vi "TLB Native Dynamic Events ver 0.13 (faulty).vi"() -> ()   [LabVIEW 2018]
uses:
  Labview Training Phase 2/Enum Controls/States for Action Engine.ctl
  TLB Type Definitions/State Type Definitions.ctl
  TLB Type Definitions/Intruction Type Definitions.ctl
  TLB Type Definitions/Encoder cluster.ctl
  TLB Type Definitions/PING CLUSTER.ctl
  <vilib>/Studica/Studica Toolkit/NavX/NavX.lvlib
  <vilib>/Studica/Studica Toolkit/Background/DIO Channel.ctl
  Underlying VI's/NavX VI/navX type def.ctl
  <vilib>/myRIO/Instrument Drivers/Utilities/Utilities.lvlib
  <vilib>/Studica/Studica Toolkit/Background/I2C Channel.ctl
  Underlying VI's/I2C Master VI/I2C MASTER Type Def.ctl
  Experimental VI's/Archived VI's/PID Movement final version Type Def.ctl
  Underlying VI's/I2C Master VI/I2C_MASTER_WRITE_NEW Type Def.ctl
  <vilib>/Studica/Studica Toolkit/NavX/TypeDefs/Flags/Z900_navX_Flags_CalibrationStatusTypeDef.ctl
  <vilib>/Studica/Studica Toolkit/NavX/TypeDefs/Flags/Z900_navX_Flags_OpStatusTypeDef.ctl
panel:
  out "Arduino I2C":errorcluster
  in  "Latch":bool
  in  "y Stepper value":u8
  in  "Arduino mode":T1
  out "Arduino Data":T2
  out "Detect?":bool
  out "Status":T5 {"OP Status" items=["INITIALIZING", "SELFTEST_IN_PROGRESS", "ERROR", "IMU_AUTOCAL_IN_PROGRESS", "NORMAL"]; "Calibration Status" items=["IMU_CAL_STATE_MASK"=3, "IMU_CAL_STATE_INPROGRESS"=0, "IMU_CAL_STATE_ACCUMULATE"=1, "IMU_CAL_STATE_COMPLETE"=2]}
  out "NavX Readings":T6
  out "TASK ENABLE":bool
  out "Rising Edge":bool
  out "Object detected?":bool
  out "navX i2C":errorcluster
  out "Speed & distance":T7
  out "State Logic":T8=enum."Startup"
  out "elements":T9[](array[typedef])
  in  "STOP TASK":bool
  in  "OK Button":bool
  in  "STOP":bool
  out "error out":errorcluster
  out "Action Queue Items":i32
  out "State Logic Queue Items":i32
  out "Action Queues items":string[](array[string])=["Hardware reset", "Software reset", ""]
  out "Action State":string
  # "TLB FRAMEWORK STATUS"
  # "System Health Status Update"
  # "Test Programme written by Calvin Loke    Dated: 28 Aug 2019\nTest Programme revised by Dr Alex See   Dated 30 Aug 2019\n\nProgramme version:   TLB Native Dynamic Events ver 0.04b.vi"
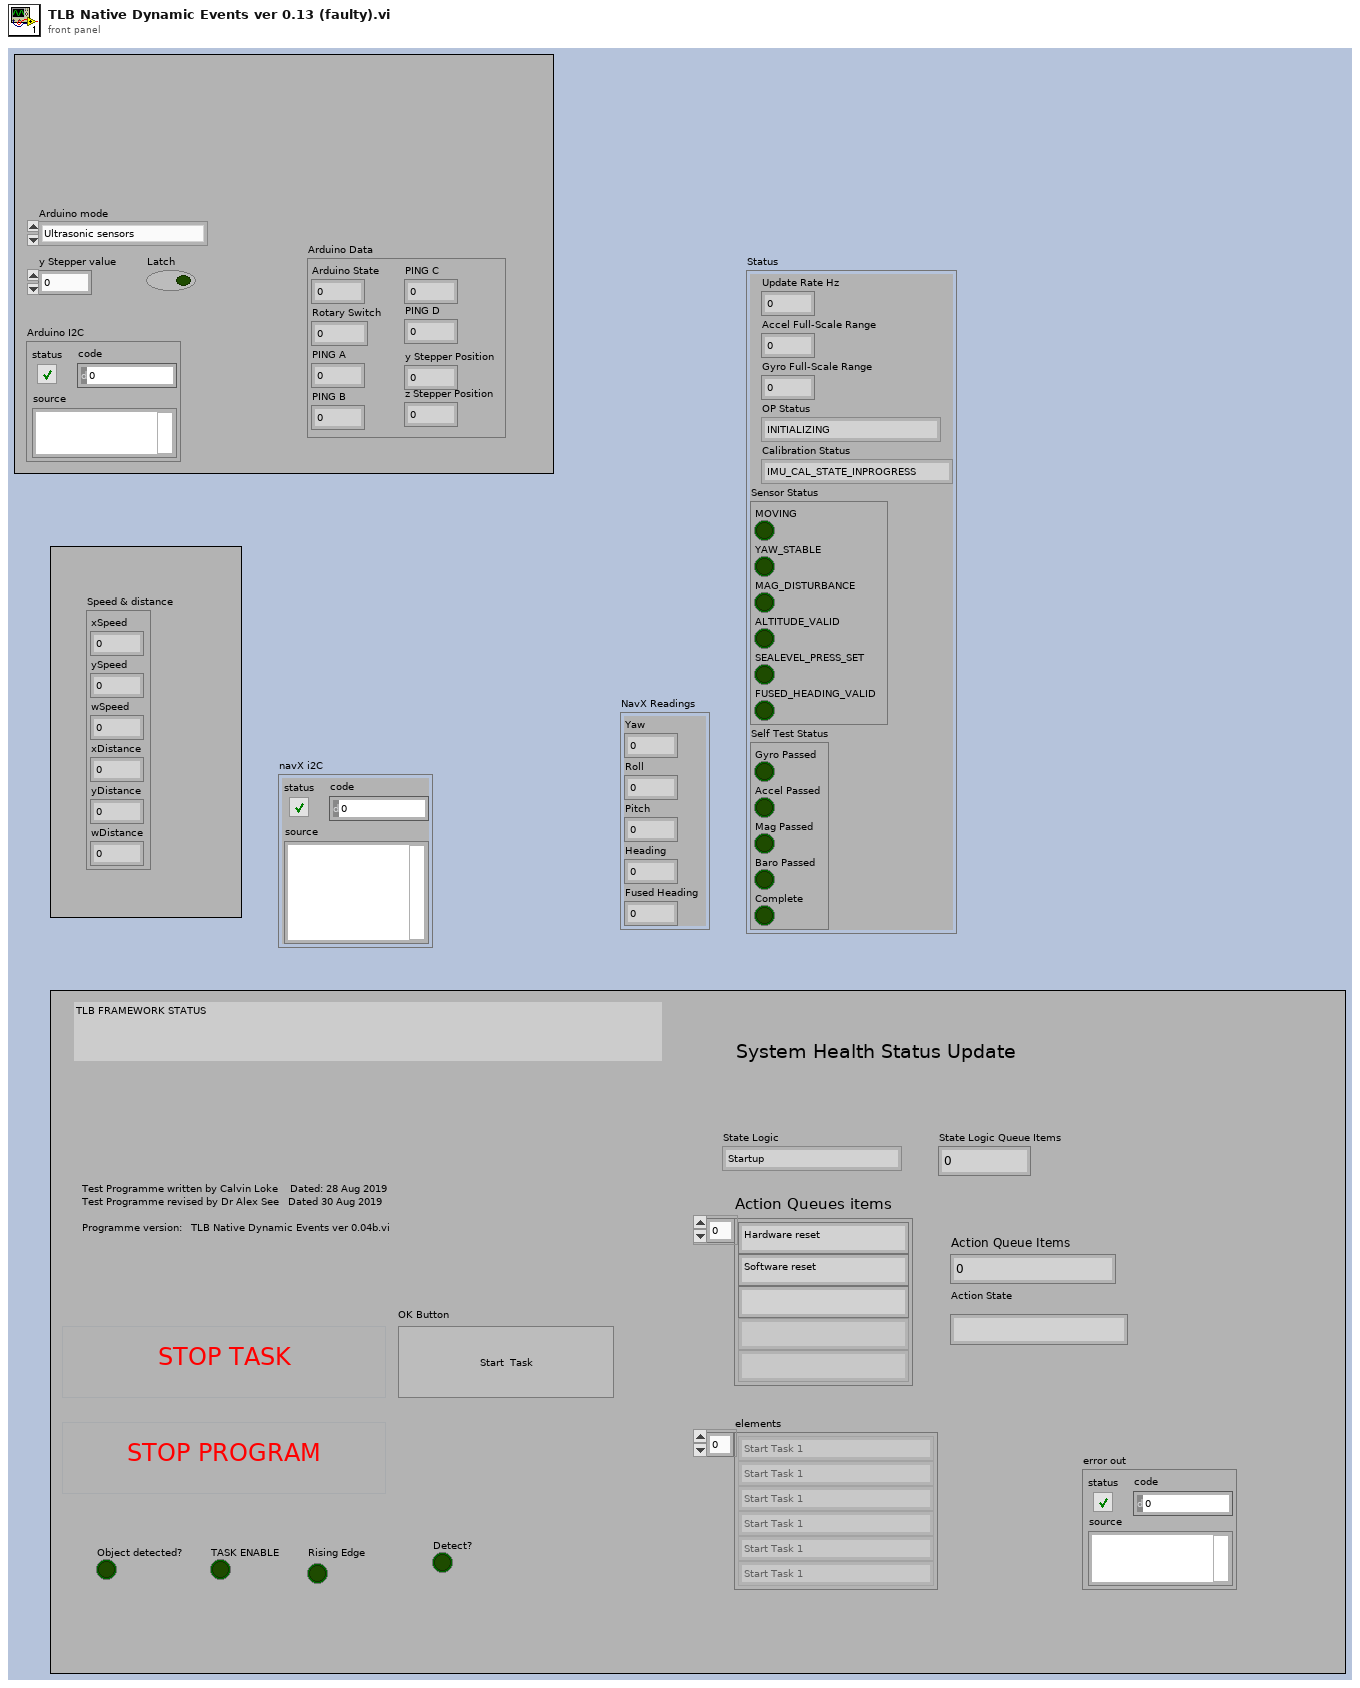
[diagram p1: front panel]
types:
  T1 = typedef "I2C_MASTER_WRITE_NEW Type Def.ctl" = enum16{"Ultrasonic sensors", "Stepper origin", "zStepper 13.3k", "zStepper 13k", "zStepper 12k", "zStepper 11k", "zStepper 10k", "zStepper 9k", "zStepper 8k", "zStepper 7k", "zStepper 6k", "zStepper 5k", "zStepper 4k", "zStepper 3k", "zStepper 2k", "zStepper 1k", "zStepper 900", "zStepper 800", "zStepper 700", "zStepper 600", "zStepper 500", "zStepper 400", "zStepper 300", "zStepper 200", "zStepper 100", "zStepper 0", "yStepper control", "Open Claw", "Close Claw", "Soft Reset"}
  T2 = cluster{"Arduino State":u8, "Rotary Switch":u8, "PING A":u8, "PING B":u8, "PING C":u8, "PING D":u8, "y Stepper Position":u8, "z Stepper Position":u8, "Data Out[8]":u8}
  T3 = typedef "NavX.lvlib/Z900_navX_Flags_OpStatusTypeDef.ctl" = u8
  T4 = typedef "NavX.lvlib/Z900_navX_Flags_CalibrationStatusTypeDef.ctl" = u8
  T5 = cluster{"Update Rate Hz":u8, "Accel Full-Scale Range":u8, "Gyro Full-Scale Range":u16, "OP Status":T3, "Calibration Status":T4, "Sensor Status":cluster{"MOVING":bool, "YAW_STABLE":bool, "MAG_DISTURBANCE":bool, "ALTITUDE_VALID":bool, "SEALEVEL_PRESS_SET":bool, "FUSED_HEADING_VALID":bool}, "Self Test Status":cluster{"Gyro Passed":bool, "Accel Passed":bool, "Mag Passed":bool, "Baro Passed":bool, "Complete":bool}}
  T6 = cluster{"Yaw":dbl, "Roll":dbl, "Pitch":dbl, "Heading":dbl, "Fused Heading":dbl}
  T7 = cluster{"xSpeed":dbl, "ySpeed":dbl, "wSpeed":dbl, "xDistance":dbl, "yDistance":dbl, "wDistance":dbl}
  T8 = typedef "State Type Definitions.ctl" = enum16{"None", "Startup", "Move to Angle", "True Stop", "Idle", "Shutdown", "Task 1A", "Task 1B", "Task 2:Raise Arm", "Task 2:Sensor Mode", "Task 2:Reverse Mode", "Task 3", "Task 4_A", "Task 4_B", "Task 4_C", "Task 4_D", "Task 5A", "Task 5B", "Task 5C", "Task 5D", "Task 5E: POSITION ARM", "Task 5F: ARM GRAB HEIGHT", "Task 5G: CLOSE CLAW", "Task 5H: RAISE ARM", "Task 6_A", "Task 6_B", "Task 7", "Task 8A: RAISE ARM", "Task 8B: MOVE TO BOX", "Task 8C: CAM BURST", "Task 8D: PROCESS IMAGE", "Task 8E: ROBOT ADJUST", "Task 8F: CAM BURST 2", "Task 8G: PROCESS IMAGE 2", "Task 8H: ARM ADJUST", "Task 8I: ARM GRAB HEIGHT", "Task 8J: CLOSE CLAW", "Task 8K: RAISE MY SWORD", "Task 9A: Raise Arm", "Task 9B: Rotate to Angle", "Task 9C: Detect Box", "Task 9D: MOVE FORWARD", "Task 9E: MOVE LEFT", "Task 9F: SCAN IMAGE", "Task 9G: PROCESS COLOUR", "Task 9H: MOVE RIGHT", "Task 9I: SCAN IMAGE", "Task 9J: PROCESS COLOUR", "Task 9K: ROTATE 90 CW", "Task 9L: MOVE FORWARD", "Task 9M: MOVE RIGHT", "Task 9N: SCAN IMAGE", "Task 9O: PROCESS COLOUR", "Task 9P: MOVE RIGHT", "Task 9Q: SCAN IMAGE", "Task 9R: PROCESS COLOUR"}
  T9 = typedef "Intruction Type Definitions.ctl" = enum16{"None", "Start Task 1", "Start Task 2", "Start Task 3", "Start Task 4", "Start Task 5", "Start Task 6", "Start Task 7", "Start Task 8 - BALL", "Start Task 8 - Gel", "Start Task 8 - Pipe", "Start Task 8 - Soap", "Start Task 9", "Start Task A", "Start Task B", "Exit"}
  T10 = typedef "States for Action Engine.ctl" = enum16{"Initialize", "Write", "Read"}
  T11 = typedef "DIO Channel.ctl" = enum16{"Not Connected", "A/DIO1", "A/DIO2", "A/DIO3", "A/DIO4", "A/DIO5", "A/DIO6", "A/DIO7", "A/DIO13", "B/DIO1", "B/DIO2", "B/DIO3", "B/DIO4", "B/DIO5", "B/DIO6", "B/DIO7", "B/DIO13", "C/DIO0", "C/DIO1", "C/DIO2", "C/DIO3", "C/DIO4", "C/DIO5", "C/DIO6", "C/DIO7"}
  T12 = typedef "PING CLUSTER.ctl" = cluster{"PING_A":u8, "PING_B":u8, "PING_C":u8, "PING_D":u8}
  T13 = typedef "Encoder cluster.ctl" = cluster{"xDistance":dbl, "yDistance":dbl, "wDistance":dbl}
  T14 = typedef "I2C Channel.ctl" = enum16{"Not Connected", "A", "B"}
  T15 = typedef "navX type def.ctl" = enum16{"Get i2C reference", "Read Values", "Zero Yaw"}
  T16 = typedef "State Type Definitions.ctl" = enum16{"None", "Startup", "Move to Angle", "True Stop", "Idle", "Shutdown", "Task 1", "Task 2:Raise Arm", "Task 2:Sensor Mode", "Task 2:Reverse Mode", "Task 3", "Task 4_A", "Task 4_B", "Task 4_C", "Task 4_D", "Task 5A: ARM CAM HEIGHT", "Task 5B: MOVE TO BOX", "Task 5C: CAM BURST", "Task 5D: PROCESS IMAGE", "Task 5E: POSITION ARM", "Task 5F: ARM GRAB HEIGHT", "Task 5G: CLOSE CLAW", "Task 5H: RAISE ARM", "Task 6_A", "Task 6_B", "Task 7", "Task 8A: RAISE ARM", "Task 8B: MOVE TO BOX", "Task 8C: CAM BURST", "Task 8D: PROCESS IMAGE", "Task 8E: ROBOT ADJUST", "Task 8F: CAM BURST 2", "Task 8G: PROCESS IMAGE 2", "Task 8H: ARM ADJUST", "Task 8I: ARM GRAB HEIGHT", "Task 8J: CLOSE CLAW", "Task 8K: RAISE MY SWORD", "Task 9A: Raise Arm", "Task 9B: Rotate to Angle", "Task 9C: Detect Box", "Task 9D: MOVE FORWARD", "Task 9E: MOVE LEFT", "Task 9F: SCAN IMAGE", "Task 9G: PROCESS COLOUR", "Task 9H: MOVE RIGHT", "Task 9I: SCAN IMAGE", "Task 9J: PROCESS COLOUR", "Task 9K: ROTATE 90 CW", "Task 9L: MOVE FORWARD", "Task 9M: MOVE RIGHT", "Task 9N: SCAN IMAGE", "Task 9O: PROCESS COLOUR", "Task 9P: MOVE RIGHT", "Task 9Q: SCAN IMAGE", "Task 9R: PROCESS COLOUR"}
  T17 = typedef "State Type Definitions.ctl" = enum16{"None", "Startup", "Move to Angle", "True Stop", "Idle", "Shutdown", "Task 1", "Task 2", "Task 3", "Task 4_A", "Task 4_B", "Task 4_C", "Task 5", "Task 6", "Task 7", "Task 8", "Task 9", "Task A", "Task B"}
  T18 = typedef "PID Movement final version Type Def.ctl" = enum16{"Init", "Front Back", "Left Right", "Rotate", "Latch", "Stop"}
  T19 = cluster{"DIO Channel":T11, "FPGA VI Reference Out":refnum<k20>}
  T20 = cluster{"I2C Ref Out":cluster{"I2C Channel":T14, "FPGA VI Reference Out":refnum<k20>}, "Connected":bool, "Slave Address (7-bit)":u8, "Registry":u8[]}
  T21 = typedef "I2C MASTER Type Def.ctl" = enum16{"Last State", "Mode 0", "Mode 1", "Mode 2", "Mode 3", "Mode 4", "Mode 5", "Mode 6", "Mode 7", "Mode 8", "Mode 9", "Mode 10"}
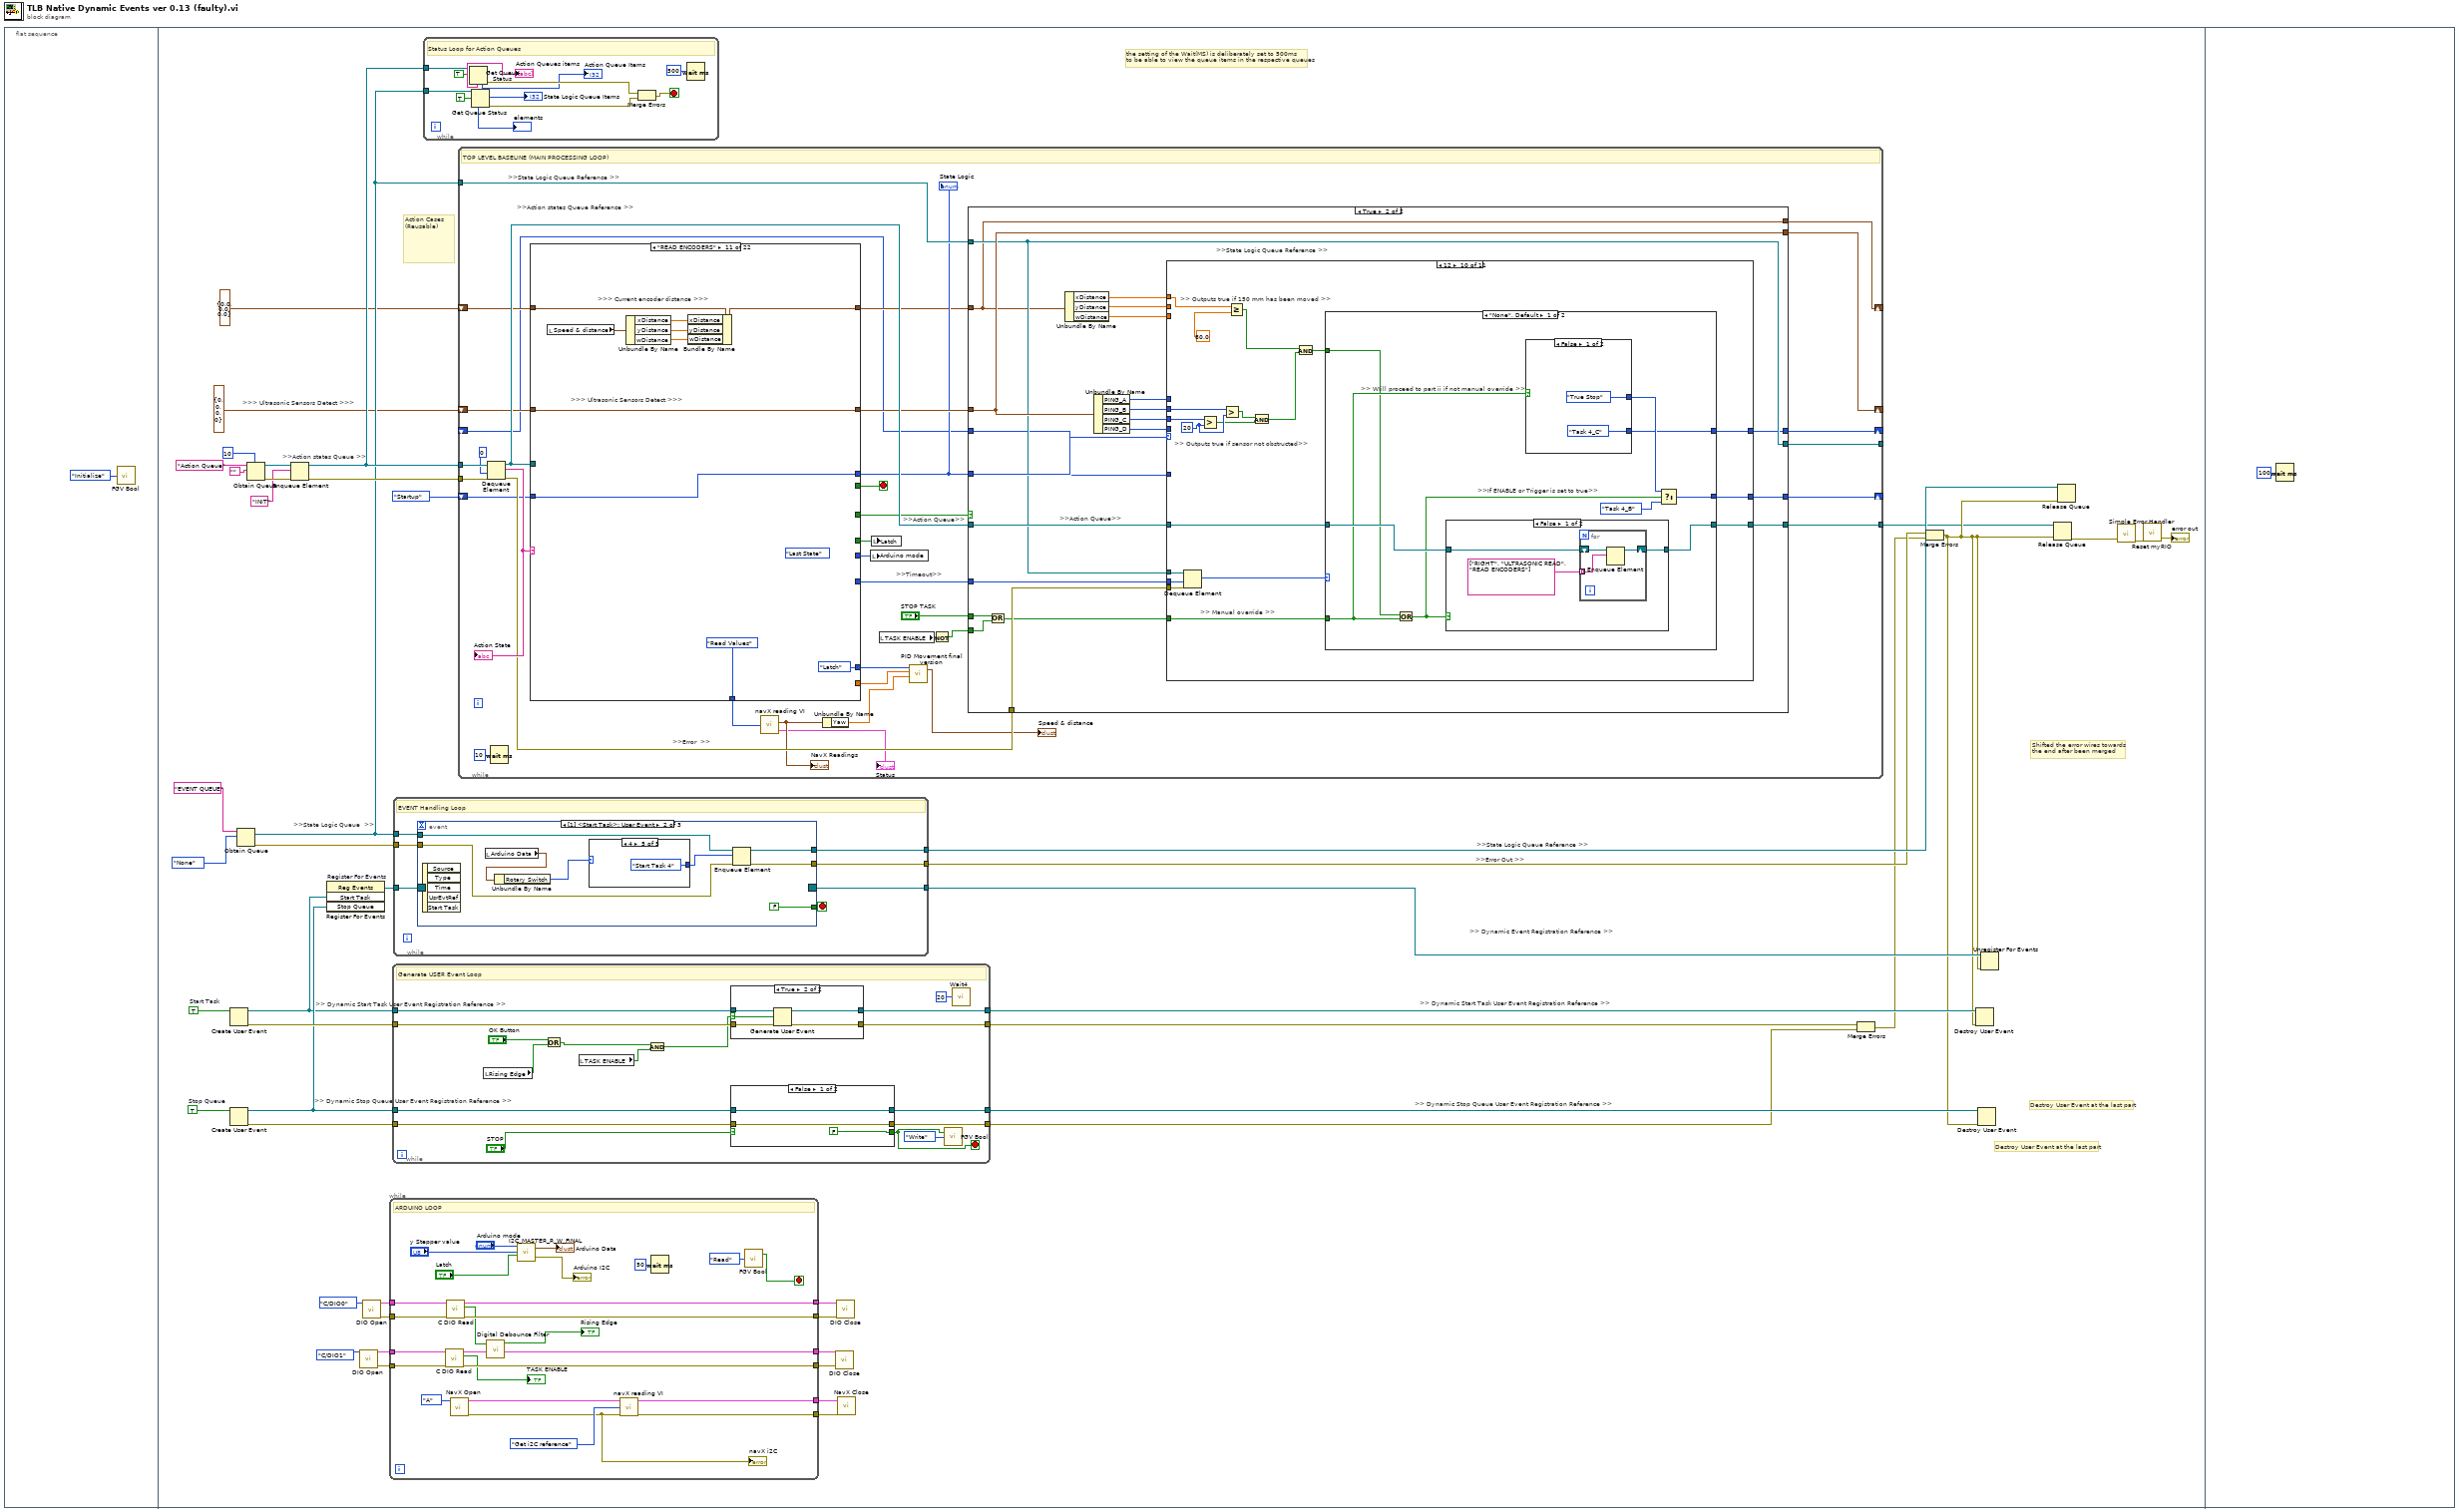
[diagram p0: block diagram]
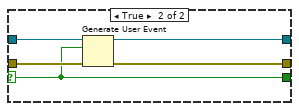
[diagram p2: hidden frame]
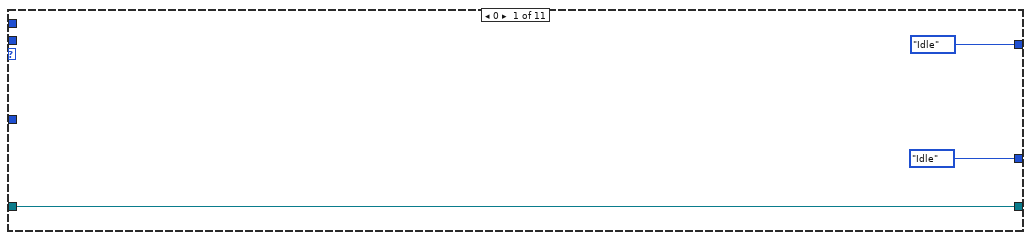
[diagram p5: hidden frame]
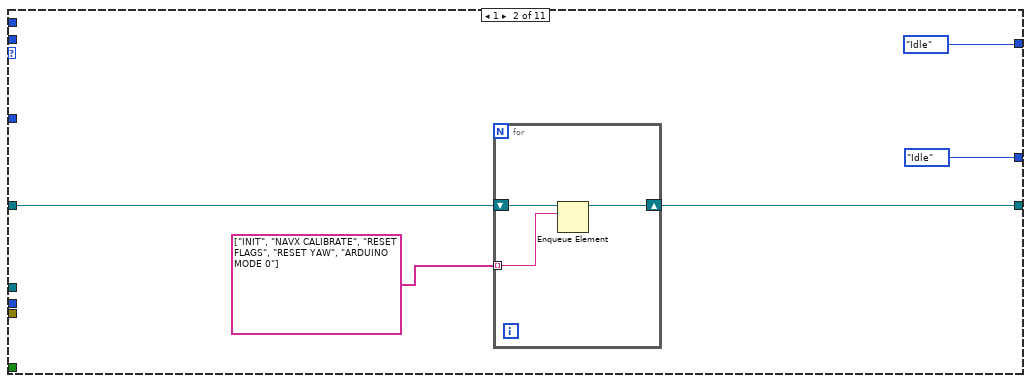
[diagram p6: hidden frame]
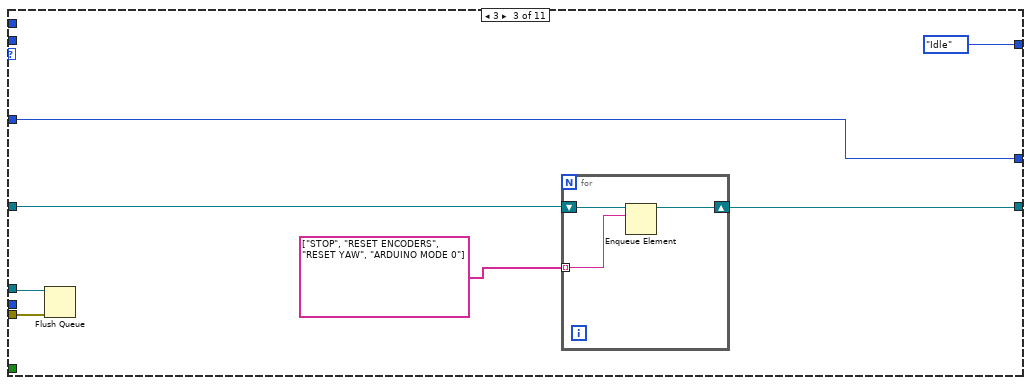
[diagram p7: hidden frame]
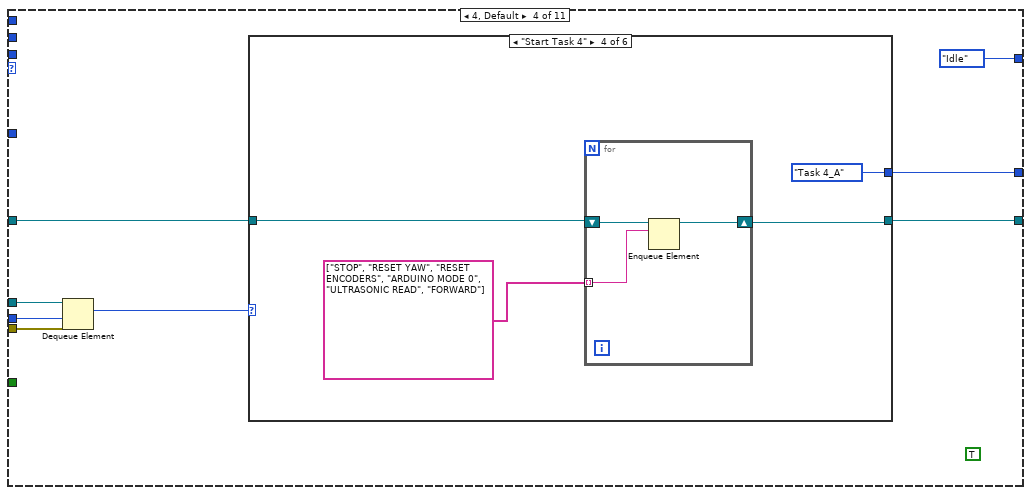
[diagram p8: hidden frame]
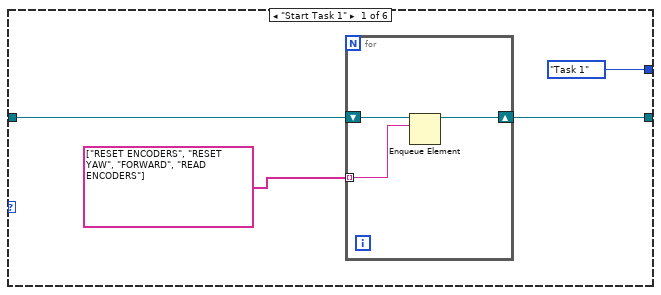
[diagram p9: hidden frame]
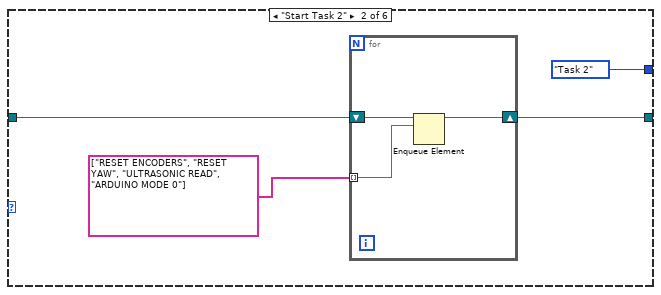
[diagram p10: hidden frame]
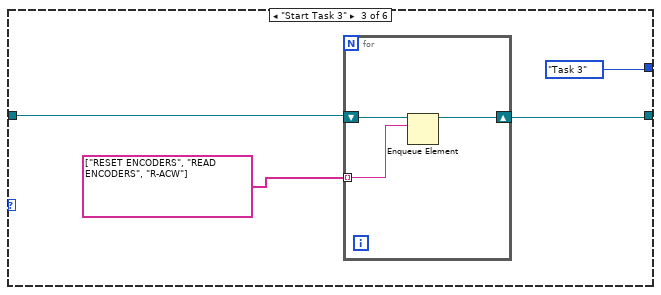
[diagram p11: hidden frame]
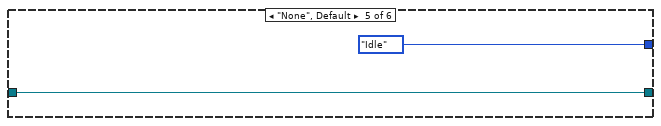
[diagram p12: hidden frame]
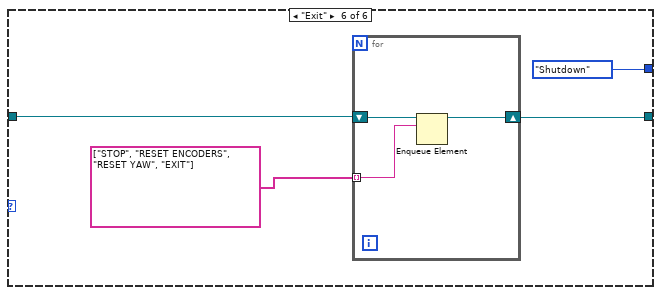
[diagram p13: hidden frame]
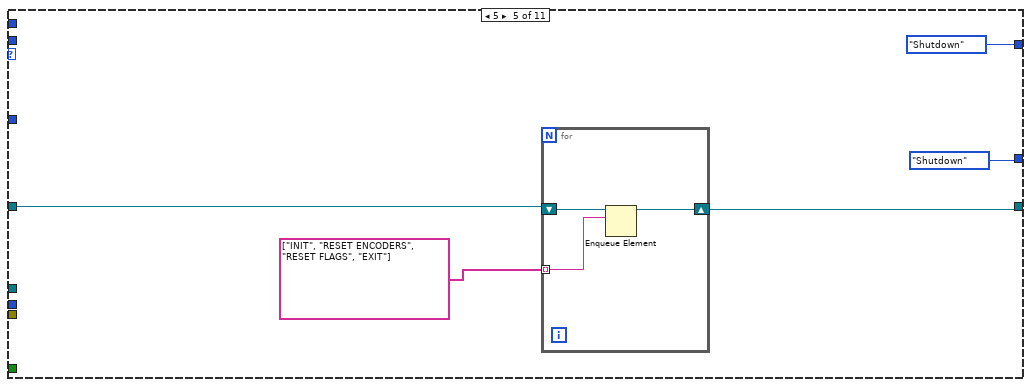
[diagram p14: hidden frame]
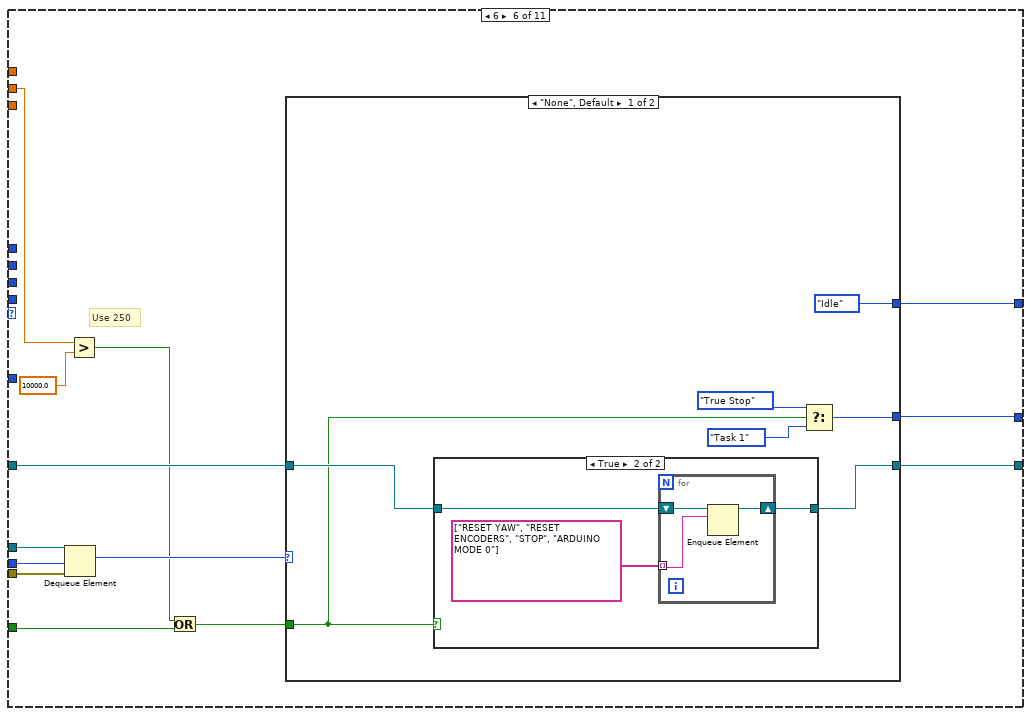
[diagram p15: hidden frame]
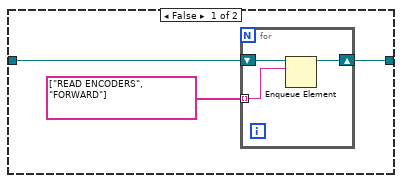
[diagram p16: hidden frame]
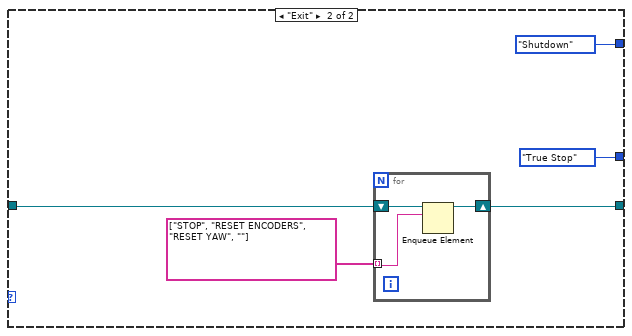
[diagram p17: hidden frame]
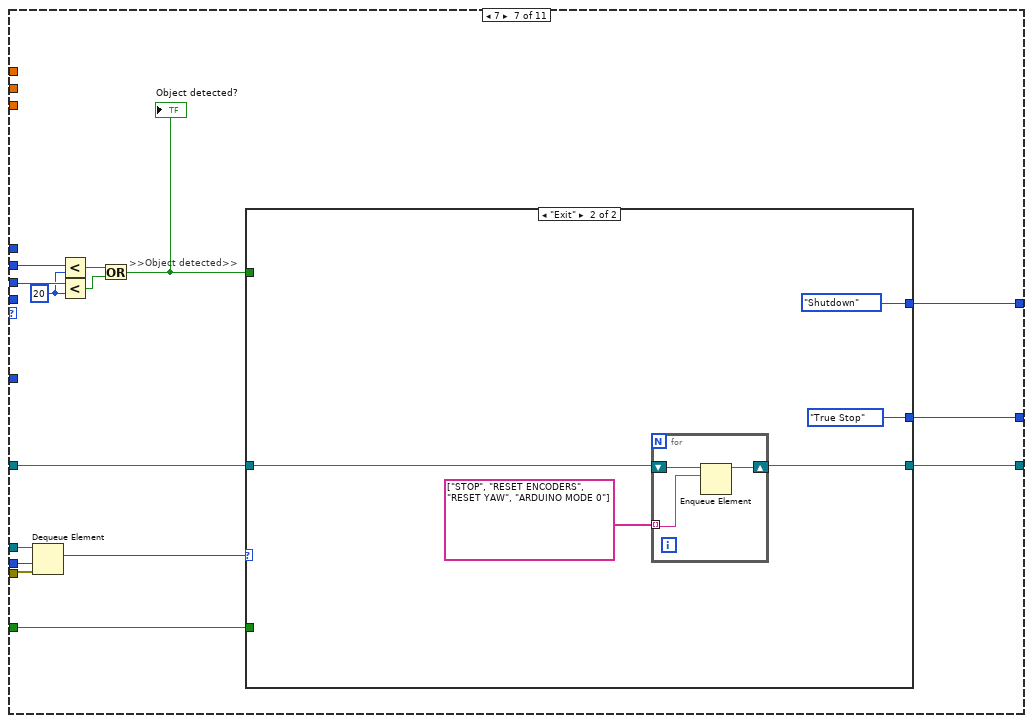
[diagram p18: hidden frame]
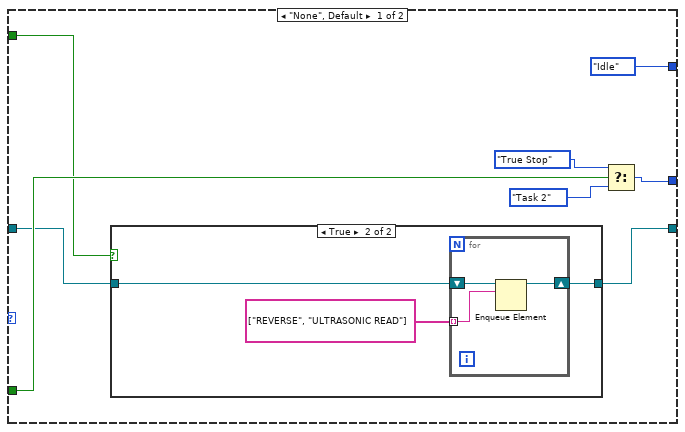
[diagram p19: hidden frame]
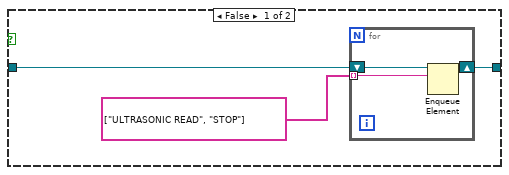
[diagram p20: hidden frame]
diagram:
  n1 = flat-sequence {
    frame #0 {
      n2 = call "FGV Bool.vi"("Init/Read/Write State"=States_for_Action_Engine."Initialize") -> ()  [unwired: 2 in, 2 out]
    }
    frame #1 {
      w48 = TRUE  # Stop Queue
      w47 = TRUE  # Start Task
      # ">>> Ultrasonic Sensors Detect >>>"
      # "the setting of the Wait(MS) is deliberately set to 500ms\nto be able to view the queue items in the respective queues"
      # "Action Cases\n(Reusable)"
      # ">>Error Out >>"
      # ">> Dynamic Stop Queue User Event Registration Reference >>"
      # ">> Dynamic Start Task User Event Registration Reference >>"
      # ">> Dynamic Stop Queue User Event Registration Reference >>"
      # ">> Dynamic Start Task User Event Registration Reference >>"
      # ">> Dynamic Event Registration Reference >>"
      # ">>Action states Queue >>"
      # ">>State Logic Queue  >>"
      # ">>State Logic Queue Reference >>"
      # "Destroy User Event at the last part"
      # "Destroy User Event at the last part"
      # "Shifted the error wires towards\nthe end after been merged"
      n3 = Create User Event(user event datatype=w47) -> (user event=w39:refnum<user-event>, error out=w44:errorcluster)  [unwired: 1 in]
      n4 = Create User Event(user event datatype=w48) -> (user event=w40:refnum<user-event>, error out=w43:errorcluster)  [unwired: 1 in]
      n5 = Obtain Queue(name (unnamed)="EVENT QUEUE", element data type=Intruction_Type_Definitions."None" ("Enum")) -> (queue out=w25:refnum<queue>, error out=w31:errorcluster)  [unwired: 3 in, 1 out]
      n6 = Obtain Queue(max queue size (-1, unlimited)=10, name (unnamed)="Action Queue", element data type="") -> (queue out=w34:refnum<queue>, error out=w30:errorcluster)  [unwired: 2 in, 1 out]
      n7 = Enqueue Element(queue=w34, element="INIT", error in (no error)=w30) -> (queue out=w26:refnum<queue>, error out=w29:errorcluster)  [unwired: 1 in, 1 out]
      n8 = register-events "Register For Events"(w39, w40) -> (reference out=w38:refnum<event-registration>)  [unwired: 2 in, 1 out]
      n9 = call <vilib>:"DIO Open.vi"("DIO Channel"=DIO_Channel."C/DIO1") -> ("error out"=w8:errorcluster, "DIO Info Out"=w9:T19)  [unwired: 9 in]
      n10 = call <vilib>:"DIO Open.vi"("DIO Channel"=DIO_Channel."C/DIO0") -> ("error out"=w13:errorcluster, "DIO Info Out"=w16:T19)  [unwired: 9 in]
      n11 = while {
        tunnel: w16 -> [w70]
        tunnel: [w69] -> w14
        tunnel: w13 -> [w68]
        tunnel: [w67] -> w12
        tunnel: [w64] -> w10
        tunnel: w9 -> [w63]
        tunnel: w8 -> [w62]
        tunnel: [w61] -> w7
        tunnel: [w58] -> w6
        tunnel: [w57] -> w5
        stop <- w72 stop-if-true
        # "ARDUINO LOOP"
        n12 = call <vilib>:"C DIO Read.vi"("error in (no error)"=w62, "DIO Info In in"=w63) -> ("error out"=w61:errorcluster, "IN"=→"TASK ENABLE":bool, "DIO Info In out"=w64:T19)  [unwired: 7 in]
        n13 = call <vilib>:"C DIO Read.vi"("error in (no error)"=w68, "DIO Info In in"=w70) -> ("error out"=w67:errorcluster, "IN"=w66:bool, "DIO Info In out"=w69:T19)  [unwired: 7 in]
        n14 = call <vilib>:"NavX Open.vi"("I2C Channel"=I2C_Channel."A") -> ("error out"=w55:errorcluster, "NavX Info"=w59:T20)  [unwired: 9 in]
        "navX i2C" <- w55
        n15 = call "Digital Debounce Filter.vi"("Boolean input"=w66) -> ("Rising Edge"=→"Rising Edge":bool)  [unwired: 1 in, 2 out]
        n16 = call "I2C_MASTER_R_W_FINAL.vi"("Latch"="Latch", "y Stepper value"="y Stepper value", "Arduino mode"="Arduino mode") -> ("error out"=→"Arduino I2C":errorcluster, "Arduino Data"=→"Arduino Data":T2)  [unwired: 1 in]
        n17 = call "navX reading VI.vi"("NavX Info In"=w59, "Mode"=navX_type_def."Get i2C reference", "error in (no error)"=w55) -> ("NavX Info Out"=w58:T20, "Error Out"=w57:errorcluster)  [unwired: 2 out]
        n18 = Wait (ms)(milliseconds to wait=u32 50) -> ()  [unwired: 1 out]
        n19 = call "FGV Bool.vi"("Init/Read/Write State"=States_for_Action_Engine."Read") -> ("Output node"=w72:bool)  [unwired: 2 in, 1 out]
      }
      n20 = while {
        tunnel: w39 -> [w102]
        tunnel: w40 -> [w101]
        tunnel: [w100] -> w46
        tunnel: [w99] -> w45
        tunnel: w44 -> [w98]
        tunnel: [w97] -> w42
        tunnel: w43 -> [w96]
        tunnel: [w95] -> w41
        stop <- w93 stop-if-true
        # "Generate USER Event Loop"
        n21 = local read "Rising Edge"() -> (w89:bool)
        n22 = Or(x="OK Button", y=w89) -> (x .or. y?=w88:bool)
        n23 = local read "TASK ENABLE"() -> (w87:bool)
        n24 = And(x=w88, y=w87) -> (x .and. y?=w86:bool)
        n25 = case shown="True" w86 {
          selector: w86 -> [_ w113]
          tunnel: w102 -> [w112 w117]
          tunnel: [w112 w116] -> w99
          tunnel: w98 -> [w111 w115]
          tunnel: [w111 w114] -> w97
          frame False {
          }
          frame True {
            n26 = Generate User Event(user event=w117, event data cluster=w113, error in=w115) -> (user event out=w116:refnum<user-event>, error out=w114:errorcluster)  [unwired: 1 in]
          }
        }
        n27 = case shown="False" "STOP" {
          selector: "STOP" -> [_ w106]
          tunnel: w101 -> [w105 w110]
          tunnel: [w105 w109] -> w100
          tunnel: w96 -> [w104 w108]
          tunnel: [w104 w107] -> w95
          tunnel: [FALSE w106] -> w93
          frame False {
          }
          frame True {
            n28 = Generate User Event(user event=w110, event data cluster=w106, error in=w108) -> (user event out=w109:refnum<user-event>, error out=w107:errorcluster)  [unwired: 1 in]
          }
        }
        n29 = call "FGV Bool.vi"("Init/Read/Write State"=States_for_Action_Engine."Write", "Input Node"=w93) -> ()  [unwired: 1 in, 2 out]
        n30 = call "Wait4"("Count(uSec)"=u32 20) -> ()  [unwired: 1 out]
      }
      n31 = while {
        tunnel: w38 -> [w660]
        tunnel: [w659] -> w37
        tunnel: w25 -> [w657]
        tunnel: [w656] -> w36
        tunnel: w31 -> [w655]
        tunnel: [w654] -> w28
        stop <- w658 stop-if-true
        # "EVENT Handling Loop"
        n32 = event shown="[1] <Start Task>: User Event" {
          selector: w660 -> [_ _ _]
          dyn-events: [_ _ _] -> w659
          timeout: _ -> [_ _ _]
          tunnel: [FALSE FALSE w685] -> w658
          tunnel: w657 -> [w665 w673 w683]
          tunnel: [w664 w672 w684] -> w656
          tunnel: w655 -> [w663 w671 w682]
          tunnel: [w662 w670 w681] -> w654
          event Timeout {
            n33 = event-data() -> ()  [unwired: 1 in, 3 out]
            n34 = Enqueue Element(queue=w665, element=Intruction_Type_Definitions."None" ("Enum"), error in (no error)=w663) -> (queue out=w664:refnum<queue>, error out=w662:errorcluster)  [unwired: 1 in, 1 out]
          }
          event User Event {
            n35 = event-data() -> ()  [unwired: 1 in, 5 out]
            n36 = local read "Arduino Data"() -> (w668:T2)
            n37 = Unbundle By Name(w668) -> ("Rotary Switch"=w667:u8)
            n38 = case shown="4" w667 {
              tunnel: [Intruction_Type_Definitions."None" ("Enum") Intruction_Type_Definitions."Start Task 1" ("Enum") Intruction_Type_Definitions."Start Task 2" ("Enum") Intruction_Type_Definitions."Start Task 3" ("Enum") Intruction_Type_Definitions."Start Task 4" ("Enum")] -> w669
              frame 0, Default {
              }
              frame 1 {
              }
              frame 2 {
              }
              frame 3 {
              }
              frame 4 {
              }
            }
            n39 = Enqueue Element(queue=w673, element=w669, error in (no error)=w671) -> (queue out=w672:refnum<queue>, error out=w670:errorcluster)  [unwired: 1 in, 1 out]
          }
          event User Event {
            n40 = event-data() -> ("Stop Queue"=w685:bool)  [unwired: 1 in, 4 out]
            n41 = Enqueue Element At Opposite End(queue=w683, element=Intruction_Type_Definitions."Exit" ("Enum"), error in (no error)=w682) -> (queue out=w684:refnum<queue>, error out=w681:errorcluster)  [unwired: 1 in, 1 out]
          }
        }
      }
      n42 = while {
        tunnel: w26 -> [w83]
        tunnel: w25 -> [w80]
        stop <- w77 stop-if-true
        # "Status Loop for Action Queues"
        n43 = Get Queue Status(queue=w83, return elements? (F)=TRUE) -> (error out=w79:errorcluster, # elements in queue=→"Action Queue Items":i32, elements=→"Action Queues items":string[])  [unwired: 1 in, 5 out]
        n44 = Get Queue Status(queue=w80, return elements? (F)=TRUE) -> (# pending remove=→"State Logic Queue Items":i32, error out=w78:errorcluster, elements=→"elements":T9[])  [unwired: 1 in, 5 out]
        n45 = Merge Errors(w79, w78) -> (w77:errorcluster)
        n46 = Wait (ms)(milliseconds to wait=u32 500) -> ()  [unwired: 1 out]
      }
      n47 = while {
        tunnel: w25 -> [w141]
        tunnel: w26 -> [w153]
        tunnel: w29 -> [w151]
        tunnel: [w150] -> _
        tunnel: [w149] -> w19
        shift-right: [w142] -> _
        shift-left: T12 {"PING_A"=0, "PING_B"=0, "PING_C"=0, "PING_D"=0} -> [w144]
        shift-right: [w135] -> _
        shift-left: State_Type_Definitions."Startup" ("Enum") -> [w138]
        shift-right: [w131] -> _
        shift-left: T13 {"xDistance"=0.0, "yDistance"=0.0, "wDistance"=0.0} -> [w133]
        shift-right: [w128] -> _
        shift-left: _ -> [w127]
        stop <- w140 stop-if-true
        # ">>Error  >>"
        # ">>Action Queue>>"
        # ">>Timeout>>"
        # ">>Action states Queue Reference >>"
        # ">>State Logic Queue Reference >>"
        # "TOP LEVEL BASELINE (MAIN PROCESSING LOOP)"
        n48 = Dequeue Element(queue=w153, timeout in ms (-1)=0, error in (no error)=w151) -> (queue out=w145:refnum<queue>, element=w152:string, error out=w146:errorcluster)  [unwired: 1 out]
        "Action State" <- w152
        n49 = Wait (ms)(milliseconds to wait=u32 10) -> ()  [unwired: 1 out]
        n50 = case shown="\"READ ENCODERS\"" w152 {
          tunnel: [_ _ _ _ _ _ _ _ _ _ _ _ _ _ _ _ 0 w630 _ _ _ _] -> w148
          tunnel: w145 -> [_ _ _ _ _ _ _ _ _ _ _ _ _ _ _ _ _ _ _ _ _ _]
          tunnel: w144 -> [w528 w532 w538 w544 w549 w554 w560 w566 w571 w573 w584 w595 w598 w608 w611 w615 w623 w631 w635 w639 w646 w653]
          tunnel: [w528 w532 w538 w544 w549 w554 w560 w566 w571 w573 w584 w596 w598 w609 w611 w615 w623 w631 w635 w639 w645 w653] -> w143
          tunnel: [TRUE TRUE _ _ _ _ _ _ _ _ _ _ _ _ _ _ _ _ _ _ _ _] -> w140
          tunnel: w138 -> [w526 w530 w537 w543 w548 w553 w559 w565 w570 w572 w583 w594 w597 w607 w610 w614 w620 w628 w634 w638 w644 w652]
          tunnel: [_ _ _ _ _ _ _ _ _ _ _ _ _ _ _ _ _ TRUE _ _ _ _] -> w137
          tunnel: [w526 w530 w537 w543 w548 w553 w559 w565 w570 w572 w583 w594 w597 w607 w610 w614 w620 w628 w634 w638 w644 w652] -> w136
          tunnel: w133 -> [w525 w529 w536 w542 w547 w552 w558 w564 w569 w574 w582 w593 w599 w606 w612 w616 w619 w627 w636 w640 w643 w651]
          tunnel: [w525 w529 w536 w542 w547 w552 w558 w564 w569 w574 w581 w593 w599 w605 w612 w616 w619 w627 w636 w640 w643 w651] -> w132
          tunnel: [_ _ 100.0 ("Speed") -50.0 ("Speed") 0.19999999999999998 ("Speed") -0.2 ("Speed") _ 0.3 ("Speed") -0.5 ("Speed") _ _ _ _ 0.0 ("Speed") _ _ _ _ _ _ _ _] -> w123
          tunnel: [_ _ navX_type_def."Read Values" ("Mode") navX_type_def."Read Values" ("Mode") _ _ navX_type_def."Read Values" ("Mode") navX_type_def."Read Values" ("Mode") _ _ navX_type_def."Read Values" ("Mode") navX_type_def."Read Values" ("Mode") _ navX_type_def."Zero Yaw" ("Mode") _ _ navX_type_def."Zero Yaw" ("Mode") navX_type_def."Read Values" ("Mode") _ _ _ navX_type_def."Zero Yaw" ("Mode")] -> w125
          tunnel: [PID_Movement_final_version_Type_Def."Init" ("Direction") _ PID_Movement_final_version_Type_Def."Front Back" ("Direction") PID_Movement_final_version_Type_Def."Left Right" ("Direction") PID_Movement_final_version_Type_Def."Rotate" ("Direction") PID_Movement_final_version_Type_Def."Rotate" ("Direction") PID_Movement_final_version_Type_Def."Stop" ("Direction") PID_Movement_final_version_Type_Def."Left Right" ("Direction") PID_Movement_final_version_Type_Def."Front Back" ("Direction") _ PID_Movement_final_version_Type_Def."Latch" ("Direction") PID_Movement_final_version_Type_Def."Latch" ("Direction") _ PID_Movement_final_version_Type_Def."Init" ("Direction") _ PID_Movement_final_version_Type_Def."Latch" ("Direction") PID_Movement_final_version_Type_Def."Latch" ("Direction") PID_Movement_final_version_Type_Def."Latch" ("Direction") _ PID_Movement_final_version_Type_Def."Init" ("Direction") PID_Movement_final_version_Type_Def."Latch" ("Direction") PID_Movement_final_version_Type_Def."Latch" ("Direction")] -> w120
          tunnel: [_ _ _ _ _ _ _ _ _ _ _ I2C_MASTER_WRITE_NEW_Type_Def."Ultrasonic sensors" ("Arduino mode") _ _ _ _ _ _ _ _ _ _] -> w119
          tunnel: [_ _ _ _ _ _ _ _ _ _ _ _ _ _ _ _ _ TRUE ("Latch") _ _ _ _] -> w118
          frame "Exit" {
            (unwired) I2C_MASTER_Type_Def."Last State" ("Arduino Mode")
          }
          frame "----Movement States----" {
            (unwired) I2C_MASTER_Type_Def."Last State" ("Arduino Mode")
          }
          frame "FORWARD" {
            (unwired) I2C_MASTER_Type_Def."Last State" ("Arduino Mode")
          }
          frame "LEFT" {
            (unwired) I2C_MASTER_Type_Def."Last State" ("Arduino Mode")
          }
          frame "R-ACW" {
            (unwired) I2C_MASTER_Type_Def."Last State" ("Arduino Mode")
          }
          frame "R-CW" {
            (unwired) I2C_MASTER_Type_Def."Last State" ("Arduino Mode")
          }
          frame "STOP" {
            (unwired) I2C_MASTER_Type_Def."Last State" ("Arduino Mode")
            n51 = Wait (ms)(milliseconds to wait=u32 200) -> ()  [unwired: 1 out]
          }
          frame "RIGHT" {
            (unwired) I2C_MASTER_Type_Def."Last State" ("Arduino Mode")
          }
          frame "REVERSE" {
            (unwired) I2C_MASTER_Type_Def."Last State" ("Arduino Mode")
          }
          frame "----SENSOR READING---- " {
            (unwired) I2C_MASTER_Type_Def."Last State" ("Arduino Mode")
          }
          frame "READ ENCODERS" {
            (unwired) I2C_MASTER_Type_Def."Last State" ("Arduino Mode")
            # ">>> Current encoder distance >>>"
            # ">>> Ultrasonic Sensors Detect >>>"
            n52 = local read "Speed & distance"() -> (w580:T7)
            n53 = Unbundle By Name(w580) -> ("xDistance"=w579:dbl, "yDistance"=w578:dbl, "wDistance"=w577:dbl)
            n54 = Bundle By Name(cluster=w582, "xDistance"=w579, "yDistance"=w578, "wDistance"=w577) -> (w581:T13)
          }
          frame "ULTRASONIC READ" {
            # "Object detection"
            n55 = local read "Arduino Data"() -> (w591:T2)
            n56 = Unbundle By Name(w591) -> ("PING A"=w590:u8, "PING B"=w589:u8, "PING C"=w588:u8, "PING D"=w587:u8)
            n57 = Bundle By Name(cluster=w595, "PING_A"=w590, "PING_B"=w589, "PING_C"=w588, "PING_D"=w587) -> (w596:T12)
          }
          frame "----SYSTEM MODES----" {
            (unwired) I2C_MASTER_Type_Def."Last State" ("Arduino Mode")
          }
          frame "INIT" {
            (unwired) I2C_MASTER_Type_Def."Last State" ("Arduino Mode")
            w602 = 0
            w604 = 0.0
            # ">>State Logic  >>"
            n58 = Bundle By Name(cluster=w608, "PING_A"=w602, "PING_B"=w602, "PING_C"=w602, "PING_D"=w602) -> (w609:T12)
            n59 = Bundle By Name(cluster=w606, "xDistance"=w604, "yDistance"=w604, "wDistance"=w604) -> (w605:T13)
          }
          frame "ARDUINO MODE 0" {
            (unwired) I2C_MASTER_Type_Def."Mode 0" ("Arduino Mode")
          }
          frame "ARDUINO MODE 1" {
            (unwired) I2C_MASTER_Type_Def."Mode 1" ("Arduino Mode")
          }
          frame "NAVX CALIBRATE" {
            (unwired) I2C_MASTER_Type_Def."Last State" ("Arduino Mode")
            # "Adds a 15 second delay to the startup process \nfor the NavX to calibrate"
            n60 = Wait (ms)(milliseconds to wait=u32 5000) -> ()  [unwired: 1 out]
          }
          frame "NO ACTION", Default {
            n61 = case shown="4" w628 {
              tunnel: [0 100] -> w630
              frame 1, Default {
              }
              frame 4 {
              }
            }
          }
          frame "----RESET CASES----" {
            (unwired) I2C_MASTER_Type_Def."Last State" ("Arduino Mode")
          }
          frame "RESET ENCODERS" {
            (unwired) I2C_MASTER_Type_Def."Last State" ("Arduino Mode")
          }
          frame "RESET FLAGS" {
            (unwired) I2C_MASTER_Type_Def."Last State" ("Arduino Mode")
            w642 = 0
            # "Resets any software variables\nand/or non-critical states"
            n62 = Wait (ms)(milliseconds to wait=u32 20) -> ()  [unwired: 1 out]
            n63 = Bundle By Name(cluster=w646, "PING_A"=w642, "PING_B"=w642, "PING_C"=w642, "PING_D"=w642) -> (w645:T12)
          }
          frame "RESET YAW" {
            (unwired) I2C_MASTER_Type_Def."Last State" ("Arduino Mode")
            n64 = Wait (ms)(milliseconds to wait=u32 100) -> ()  [unwired: 1 out]
          }
        }
        "State Logic" <- w136
        n65 = call "navX reading VI.vi"("Mode"=w125) -> ("NavX Readings"=w126:T6, "Status"=→"Status":T5)  [unwired: 2 in, 2 out]
        "NavX Readings" <- w126
        n66 = Unbundle By Name(w126) -> ("Yaw"=w122:dbl)
        n67 = local write "Arduino mode"(w119) -> ()
        n68 = local write "Latch"(w118) -> ()
        n69 = local read "TASK ENABLE"() -> (w130:bool)
        n70 = call "PID Movement final version.vi"("Yaw"=w122, "Speed"=w123, "Direction"=w120) -> ("Speed & distance"=→"Speed & distance":T7)  [unwired: 1 in, 1 out]
        n71 = Not(x=w130) -> (.not. x?=w129:bool)
        n72 = case shown="True" w137 {
          tunnel: w141 -> [w159 w175]
          tunnel: w145 -> [w155 w177]
          tunnel: [w159 w175] -> w150
          tunnel: [w155 w178] -> w149
          tunnel: w146 -> [_ w173]
          tunnel: w148 -> [_ w174]
          tunnel: w143 -> [w158 w180]
          tunnel: [w158 w180] -> w142
          tunnel: "STOP TASK" -> [_ w163]
          tunnel: w136 -> [w157 w179]
          tunnel: [w157 w176] -> w135
          tunnel: w132 -> [w156 w169]
          tunnel: [w156 w169] -> w131
          tunnel: w129 -> [_ w164]
          tunnel: [w154 w161] -> w128
          tunnel: w127 -> [w154 w160]
          frame False {
          }
          frame True {
            # ">>Action Queue>>"
            # ">>State Logic Queue Reference >>"
            n73 = Or(x=w163, y=w164) -> (x .or. y?=w162:bool)
            n74 = Unbundle By Name(w169) -> ("xDistance"=w166:dbl, "yDistance"=w167:dbl, "wDistance"=w168:dbl)
            n75 = Unbundle By Name(w180) -> ("PING_A"=w172:u8, "PING_B"=w171:u8, "PING_C"=w170:u8, "PING_D"=w165:u8)
            n76 = case shown="12" w179 {
              tunnel: [w182 w185 w196 w203 w248 w260 w296 w342 w386 w443 w480] -> w178
              tunnel: w177 -> [w182 w188 w197 w206 w250 w261 w297 w343 w392 w436 w484]
              tunnel: [State_Type_Definitions."Idle" ("Enum") State_Type_Definitions."Idle" ("Enum") w192 w205 State_Type_Definitions."Shutdown" ("Enum") w262 w299 w341 w387 w442 w481] -> w176
              tunnel: w175 -> [_ _ w195 w209 _ w267 w309 w350 w391 w440 w485]
              tunnel: w174 -> [_ _ _ w208 _ w266 w308 w349 w390 w439 w477]
              tunnel: w173 -> [_ _ w194 w204 _ w265 w307 w348 w389 w438 w476]
              tunnel: w162 -> [_ _ _ _ _ w259 w298 w345 w385 w441 w482]
              tunnel: w172 -> [_ _ _ _ _ _ _ _ _ _ _]
              tunnel: w171 -> [_ _ _ _ _ _ w305 _ w383 w431 w487]
              tunnel: w170 -> [_ _ _ _ _ _ w304 _ w384 w432 w486]
              tunnel: w168 -> [_ _ _ _ _ _ _ w347 _ _ _]
              tunnel: w167 -> [_ _ _ _ _ w258 _ _ _ _ _]
              tunnel: w166 -> [_ _ _ _ _ _ _ _ _ w427 _]
              tunnel: w165 -> [_ _ _ _ _ _ _ _ _ _ _]
              tunnel: [State_Type_Definitions."Idle" ("Enum") State_Type_Definitions."Idle" ("Enum") State_Type_Definitions."Idle" ("Enum") State_Type_Definitions."Idle" ("Enum") State_Type_Definitions."Shutdown" ("Enum") w255 w295 w338 w378 w426 w479] -> w161
              tunnel: w160 -> [_ _ w192 _ _ _ _ _ _ _ _]
              frame 0 {
              }
              frame 1 {
                n77 = for {
                  shift-right: [w191] -> w185
                  shift-left: w188 -> [w190]
                  tunnel: string[] ["INIT", "NAVX CALIBRATE", "RESET FLAGS", "RESET YAW", "ARDUINO MODE 0"] -> [w189] mode=indexing
                  n78 = Enqueue Element(queue=w190, element=w189) -> (queue out=w191:refnum<queue>)  [unwired: 2 in, 2 out]
                }
              }
              frame 3 {
                n79 = Flush Queue(queue=w195, error in (no error)=w194) -> ()  [unwired: 3 out]
                n80 = for {
                  shift-right: [w201] -> w196
                  shift-left: w197 -> [w200]
                  tunnel: string[] ["STOP", "RESET ENCODERS", "RESET YAW", "ARDUINO MODE 0"] -> [w199] mode=indexing
                  n81 = Enqueue Element(queue=w200, element=w199) -> (queue out=w201:refnum<queue>)  [unwired: 2 in, 2 out]
                }
              }
              frame 4, Default {
                (unwired) TRUE ("Green LED")
                n82 = Dequeue Element(queue=w209, timeout in ms (-1)=w208, error in (no error)=w204) -> (element=w207:T9)  [unwired: 3 out]
                n83 = case shown="\"Start Task 4\"" w207 {
                  tunnel: [w211 w218 w225 w232 w239 w241] -> w203
                  tunnel: w206 -> [w212 w219 w226 w233 w239 w242]
                  tunnel: [State_Type_Definitions."Task 1" ("Enum") State_Type_Definitions."Task 2" ("Enum") State_Type_Definitions."Task 3" ("Enum") State_Type_Definitions."Task 4_A" ("Enum") State_Type_Definitions."Idle" ("Enum") State_Type_Definitions."Shutdown" ("Enum")] -> w205
                  frame "Start Task 1" {
                    n84 = for {
                      shift-right: [w216] -> w211
                      shift-left: w212 -> [w215]
                      tunnel: string[] ["RESET ENCODERS", "RESET YAW", "FORWARD", "READ ENCODERS"] -> [w214] mode=indexing
                      n85 = Enqueue Element(queue=w215, element=w214) -> (queue out=w216:refnum<queue>)  [unwired: 2 in, 2 out]
                    }
                  }
                  frame "Start Task 2" {
                    n86 = for {
                      shift-right: [w223] -> w218
                      shift-left: w219 -> [w222]
                      tunnel: string[] ["RESET ENCODERS", "RESET YAW", "ULTRASONIC READ", "ARDUINO MODE 0"] -> [w221] mode=indexing
                      n87 = Enqueue Element(queue=w222, element=w221) -> (queue out=w223:refnum<queue>)  [unwired: 2 in, 2 out]
                    }
                  }
                  frame "Start Task 3" {
                    n88 = for {
                      shift-right: [w230] -> w225
                      shift-left: w226 -> [w229]
                      tunnel: string[] ["RESET ENCODERS", "READ ENCODERS", "R-ACW"] -> [w228] mode=indexing
                      n89 = Enqueue Element(queue=w229, element=w228) -> (queue out=w230:refnum<queue>)  [unwired: 2 in, 2 out]
                    }
                  }
                  frame "Start Task 4" {
                    n90 = for {
                      shift-right: [w237] -> w232
                      shift-left: w233 -> [w236]
                      tunnel: string[] ["STOP", "RESET YAW", "RESET ENCODERS", "ARDUINO MODE 0", "ULTRASONIC READ", "FORWARD"] -> [w235] mode=indexing
                      n91 = Enqueue Element(queue=w236, element=w235) -> (queue out=w237:refnum<queue>)  [unwired: 2 in, 2 out]
                    }
                  }
                  frame "None", Default {
                  }
                  frame "Exit" {
                    n92 = for {
                      shift-right: [w246] -> w241
                      shift-left: w242 -> [w245]
                      tunnel: string[] ["STOP", "RESET ENCODERS", "RESET YAW", "EXIT"] -> [w244] mode=indexing
                      n93 = Enqueue Element(queue=w245, element=w244) -> (queue out=w246:refnum<queue>)  [unwired: 2 in, 2 out]
                    }
                  }
                }
              }
              frame 5 {
                n94 = for {
                  shift-right: [w254] -> w248
                  shift-left: w250 -> [w253]
                  tunnel: string[] ["INIT", "RESET ENCODERS", "RESET FLAGS", "EXIT"] -> [w252] mode=indexing
                  n95 = Enqueue Element(queue=w253, element=w252) -> (queue out=w254:refnum<queue>)  [unwired: 2 in, 2 out]
                }
              }
              frame 6 {
                # "Use 250"
                n96 = Dequeue Element(queue=w267, timeout in ms (-1)=w266, error in (no error)=w265) -> (element=w264:T9)  [unwired: 3 out]
                n97 = Greater?(x=w258, y=10000.0) -> (0:w256:bool)
                n98 = Or(x=w256, y=w259) -> (x .or. y?=w263:bool)
                n99 = case shown="\"None\", Default" w264 {
                  tunnel: w263 -> [w270 _]
                  tunnel: [w274 State_Type_Definitions."True Stop" ("Enum")] -> w262
                  tunnel: w261 -> [w271 w289]
                  tunnel: [w269 w288] -> w260
                  tunnel: [State_Type_Definitions."Idle" ("Enum") State_Type_Definitions."Shutdown" ("Enum")] -> w255
                  frame "None", Default {
                    n100 = case shown="True" w270 {
                      tunnel: w271 -> [w277 w283]
                      tunnel: [w276 w281] -> w269
                      frame False {
                        n101 = for {
                          shift-right: [w279] -> w276
                          shift-left: w277 -> [w280]
                          tunnel: string[] ["READ ENCODERS", "FORWARD"] ("element") -> [w278] mode=indexing
                          n102 = Enqueue Element(queue=w280, element=w278) -> (queue out=w279:refnum<queue>)  [unwired: 2 in, 2 out]
                        }
                      }
                      frame True {
                        n103 = for {
                          shift-right: [w285] -> w281
                          shift-left: w283 -> [w286]
                          tunnel: string[] ["RESET YAW", "RESET ENCODERS", "STOP", "ARDUINO MODE 0"] -> [w284] mode=indexing
                          n104 = Enqueue Element(queue=w286, element=w284) -> (queue out=w285:refnum<queue>)  [unwired: 2 in, 2 out]
                        }
                      }
                    }
                    n105 = Select(t=State_Type_Definitions."True Stop" ("Enum"), s=w270, f=State_Type_Definitions."Task 1" ("Enum")) -> (s? t:f=w274:u16)
                  }
                  frame "Exit" {
                    n106 = for {
                      shift-right: [w293] -> w288
                      shift-left: w289 -> [w294]
                      tunnel: string[] ["STOP", "RESET ENCODERS", "RESET YAW", ""] -> [w292] mode=indexing
                      n107 = Enqueue Element(queue=w294, element=w292) -> (queue out=w293:refnum<queue>)  [unwired: 2 in, 2 out]
                    }
                  }
                }
              }
              frame 7 {
                w303 = u16 20 ("y")
                # ">>Object detected>>"
                n108 = Dequeue Element(queue=w309, timeout in ms (-1)=w308, error in (no error)=w307) -> (element=w306:T9)  [unwired: 3 out]
                n109 = Less?(x=w305, y=w303) -> (x < y?=w302:bool)
                n110 = Less?(x=w304, y=w303) -> (x < y?=w301:bool)
                n111 = Or(x=w302, y=w301) -> (x .or. y?=w300:bool)
                "Object detected?" <- w300
                n112 = case shown="\"Exit\"" w306 {
                  tunnel: w300 -> [w313 _]
                  tunnel: [w315 State_Type_Definitions."True Stop" ("Enum")] -> w299
                  tunnel: w298 -> [w314 _]
                  tunnel: w297 -> [w312 w332]
                  tunnel: [w311 w333] -> w296
                  tunnel: [State_Type_Definitions."Idle" ("Enum") State_Type_Definitions."Shutdown" ("Enum")] -> w295
                  frame "None", Default {
                    n113 = case shown="True" w313 {
                      tunnel: w312 -> [w319 w326]
                      tunnel: [w320 w325] -> w311
                      frame False {
                        n114 = for {
                          tunnel: string[] ["ULTRASONIC READ", "STOP"] ("element") -> [w321] mode=indexing
                          shift-right: [w323] -> w320
                          shift-left: w319 -> [w322]
                          n115 = Enqueue Element(queue=w322, element=w321) -> (queue out=w323:refnum<queue>)  [unwired: 2 in, 2 out]
                        }
                      }
                      frame True {
                        n116 = for {
                          shift-right: [w328] -> w325
                          shift-left: w326 -> [w329]
                          tunnel: string[] ["REVERSE", "ULTRASONIC READ"] -> [w327] mode=indexing
                          n117 = Enqueue Element(queue=w329, element=w327) -> (queue out=w328:refnum<queue>)  [unwired: 2 in, 2 out]
                        }
                      }
                    }
                    n118 = Select(t=State_Type_Definitions."True Stop" ("Enum"), s=w314, f=State_Type_Definitions."Task 2" ("Enum")) -> (s? t:f=w315:u16)
                  }
                  frame "Exit" {
                    n119 = for {
                      shift-right: [w336] -> w333
                      shift-left: w332 -> [w337]
                      tunnel: string[] ["STOP", "RESET ENCODERS", "RESET YAW", "ARDUINO MODE 0"] -> [w335] mode=indexing
                      n120 = Enqueue Element(queue=w337, element=w335) -> (queue out=w336:refnum<queue>)  [unwired: 2 in, 2 out]
                    }
                  }
                }
              }
              frame 10 {
                n121 = Dequeue Element(queue=w350, timeout in ms (-1)=w349, error in (no error)=w348) -> (element=w339:T9)  [unwired: 3 out]
                n122 = Greater?(x=w347, y=150.0) -> (0:w344:bool)
                n123 = Or(x=w344, y=w345) -> (x .or. y?=w340:bool)
                n124 = case shown="\"Exit\"" w339 {
                  tunnel: w340 -> [w353 _]
                  tunnel: [w357 State_Type_Definitions."True Stop" ("Enum")] -> w341
                  tunnel: w343 -> [w354 w373]
                  tunnel: [w352 w372] -> w342
                  tunnel: [State_Type_Definitions."Idle" ("Enum") State_Type_Definitions."Shutdown" ("Enum")] -> w338
                  frame "None", Default {
                    n125 = case shown="False" w353 {
                      tunnel: w354 -> [w360 w366]
                      tunnel: [w359 w364] -> w352
                      frame False {
                        n126 = for {
                          shift-right: [w362] -> w359
                          shift-left: w360 -> [w363]
                          tunnel: string[] ["READ ENCODERS", "R-ACW"] ("element") -> [w361] mode=indexing
                          n127 = Enqueue Element(queue=w363, element=w361) -> (queue out=w362:refnum<queue>)  [unwired: 2 in, 2 out]
                        }
                      }
                      frame True {
                        n128 = for {
                          shift-right: [w368] -> w364
                          shift-left: w366 -> [w369]
                          tunnel: string[] ["RESET YAW", "RESET ENCODERS", "STOP", "ARDUINO MODE 0"] -> [w367] mode=indexing
                          n129 = Enqueue Element(queue=w369, element=w367) -> (queue out=w368:refnum<queue>)  [unwired: 2 in, 2 out]
                        }
                      }
                    }
                    n130 = Select(t=State_Type_Definitions."True Stop" ("Enum"), s=w353, f=State_Type_Definitions."Task 3" ("Enum")) -> (s? t:f=w357:T8)
                  }
                  frame "Exit" {
                    n131 = for {
                      shift-right: [w376] -> w372
                      shift-left: w373 -> [w377]
                      tunnel: string[] ["STOP", "RESET ENCODERS", "RESET YAW", ""] -> [w375] mode=indexing
                      n132 = Enqueue Element(queue=w377, element=w375) -> (queue out=w376:refnum<queue>)  [unwired: 2 in, 2 out]
                    }
                  }
                }
              }
              frame 11 {
                w382 = 50
                # ">> Outputs true if object detected >>"
                # ">> Manual override >>"
                n133 = Dequeue Element(queue=w391, timeout in ms (-1)=w390, error in (no error)=w389) -> (element=w388:T9)  [unwired: 3 out]
                n134 = Less?(x=w384, y=w382) -> (x < y?=w380:bool)
                n135 = Less?(x=w383, y=w382) -> (x < y?=w381:bool)
                n136 = And(x=w381, y=w380) -> (x .and. y?=w379:bool)
                "Detect?" <- w379
                n137 = case shown="\"None\", Default" w388 {
                  tunnel: [w401 State_Type_Definitions."True Stop" ("Enum")] -> w387
                  tunnel: [w399 w420] -> w386
                  tunnel: w392 -> [w398 _]
                  tunnel: w385 -> [w396 _]
                  tunnel: w379 -> [w394 _]
                  tunnel: [w393 State_Type_Definitions."Shutdown" ("Enum")] -> w378
                  frame "None", Default {
                    # ">> WIill proceed to part ii if not manual override >>"
                    # ">>If ENABLE or Trigger is set to true>>"
                    n138 = Or(x=w394, y=w396) -> (x .or. y?=w395:bool)
                    n139 = case shown="False" w395 {
                      tunnel: [w408 w413] -> w399
                      tunnel: w398 -> [w406 w412]
                      frame False {
                        n140 = for {
                          shift-right: [w410] -> w408
                          shift-left: w406 -> [w411]
                          tunnel: string[] ["FORWARD", "ULTRASONIC READ", ""] ("element") -> [w409] mode=indexing
                          n141 = Enqueue Element(queue=w411, element=w409) -> (queue out=w410:refnum<queue>)  [unwired: 2 in, 2 out]
                        }
                      }
                      frame True {
                        n142 = for {
                          shift-right: [w416] -> w413
                          shift-left: w412 -> [w417]
                          tunnel: string[] ["STOP", "RESET ENCODERS", "RESET YAW", "ARDUINO MODE 0"] -> [w415] mode=indexing
                          n143 = Enqueue Element(queue=w417, element=w415) -> (queue out=w416:refnum<queue>)  [unwired: 2 in, 2 out]
                        }
                      }
                    }
                    n144 = case shown="False" w396 {
                      tunnel: [State_Type_Definitions."True Stop" ("Enum") State_Type_Definitions."True Stop" ("Enum")] -> w397
                      tunnel: [State_Type_Definitions."Task 4_B" ("Enum") State_Type_Definitions."Idle" ("Enum")] -> w393
                      frame False {
                      }
                      frame True {
                      }
                    }
                    n145 = Select(t=w397, s=w395, f=State_Type_Definitions."Task 4_A" ("Enum")) -> (s? t:f=w401:T8)
                  }
                  frame "Exit" {
                    n146 = for {
                      shift-right: [w423] -> w420
                      shift-left: _ -> [w424]
                      tunnel: string[] ["STOP", "RESET ENCODERS", "RESET YAW", ""] -> [w422] mode=indexing
                      n147 = Enqueue Element(queue=w424, element=w422) -> (queue out=w423:refnum<queue>)  [unwired: 2 in, 2 out]
                    }
                  }
                }
              }
              frame 12 {
                w435 = 20
                # ">> Outputs true if 150 mm has been moved >>"
                # ">> Outputs true if sensor not obstructed>>"
                # ">> Manual override >>"
                n148 = Dequeue Element(queue=w440, timeout in ms (-1)=w439, error in (no error)=w438) -> (element=w437:T9)  [unwired: 3 out]
                n149 = Greater?(x=w432, y=w435) -> (0:w433:bool)
                n150 = Greater?(x=w431, y=w435) -> (0:w434:bool)
                n151 = Greater Or Equal?(x=w427, y=80.0) -> (x >= y?=w429:bool)
                n152 = And(x=w434, y=w433) -> (x .and. y?=w428:bool)
                n153 = And(x=w429, y=w428) -> (x .and. y?=w425:bool)
                n154 = case shown="\"None\", Default" w437 {
                  tunnel: [w452 State_Type_Definitions."True Stop" ("Enum")] -> w442
                  tunnel: [w450 w471] -> w443
                  tunnel: w436 -> [w449 _]
                  tunnel: w441 -> [w447 _]
                  tunnel: w425 -> [w445 _]
                  tunnel: [w444 State_Type_Definitions."Shutdown" ("Enum")] -> w426
                  frame "None", Default {
                    # ">> WIill proceed to part ii if not manual override >>"
                    # ">>If ENABLE or Trigger is set to true>>"
                    n155 = Or(x=w445, y=w447) -> (x .or. y?=w446:bool)
                    n156 = case shown="False" w446 {
                      tunnel: [w459 w464] -> w450
                      tunnel: w449 -> [w457 w463]
                      frame False {
                        n157 = for {
                          shift-right: [w461] -> w459
                          shift-left: w457 -> [w462]
                          tunnel: string[] ["RIGHT", "ULTRASONIC READ", "READ ENCODERS"] ("element") -> [w460] mode=indexing
                          n158 = Enqueue Element(queue=w462, element=w460) -> (queue out=w461:refnum<queue>)  [unwired: 2 in, 2 out]
                        }
                      }
                      frame True {
                        n159 = for {
                          shift-right: [w467] -> w464
                          shift-left: w463 -> [w468]
                          tunnel: string[] ["STOP", "RESET ENCODERS", "RESET YAW", "ARDUINO MODE 0"] -> [w466] mode=indexing
                          n160 = Enqueue Element(queue=w468, element=w466) -> (queue out=w467:refnum<queue>)  [unwired: 2 in, 2 out]
                        }
                      }
                    }
                    n161 = case shown="False" w447 {
                      tunnel: [State_Type_Definitions."True Stop" ("Enum") State_Type_Definitions."True Stop" ("Enum")] -> w448
                      tunnel: [State_Type_Definitions."Task 4_C" ("Enum") State_Type_Definitions."Idle" ("Enum")] -> w444
                      frame False {
                      }
                      frame True {
                      }
                    }
                    n162 = Select(t=w448, s=w446, f=State_Type_Definitions."Task 4_B" ("Enum")) -> (s? t:f=w452:T8)
                  }
                  frame "Exit" {
                    n163 = for {
                      shift-right: [w474] -> w471
                      shift-left: _ -> [w475]
                      tunnel: string[] ["STOP", "RESET ENCODERS", "RESET YAW", ""] -> [w473] mode=indexing
                      n164 = Enqueue Element(queue=w475, element=w473) -> (queue out=w474:refnum<queue>)  [unwired: 2 in, 2 out]
                    }
                  }
                }
              }
              frame 13 {
                w490 = 30
                # ">> Outputs true if object detected >>"
                # ">> Manual override >>"
                n165 = Dequeue Element(queue=w485, timeout in ms (-1)=w477, error in (no error)=w476) -> (element=w478:T9)  [unwired: 3 out]
                n166 = Less?(x=w486, y=w490) -> (x < y?=w488:bool)
                n167 = Less?(x=w487, y=w490) -> (x < y?=w489:bool)
                n168 = And(x=w489, y=w488) -> (x .and. y?=w483:bool)
                n169 = case shown="\"None\", Default" w478 {
                  tunnel: [w499 State_Type_Definitions."True Stop" ("Enum")] -> w481
                  tunnel: [w497 w519] -> w480
                  tunnel: w484 -> [w496 w516]
                  tunnel: w482 -> [w494 _]
                  tunnel: w483 -> [w492 _]
                  tunnel: [w491 State_Type_Definitions."Shutdown" ("Enum")] -> w479
                  frame "None", Default {
                    # ">> WIill proceed to part ii if not manual override >>"
                    # ">>If ENABLE or Trigger is set to true>>"
                    n170 = Or(x=w492, y=w494) -> (x .or. y?=w493:bool)
                    n171 = case shown="False" w493 {
                      tunnel: [w506 w511] -> w497
                      tunnel: w496 -> [w504 w510]
                      frame False {
                        n172 = for {
                          shift-right: [w508] -> w506
                          shift-left: w504 -> [w509]
                          tunnel: string[] ["FORWARD", "ULTRASONIC READ", ""] ("element") -> [w507] mode=indexing
                          n173 = Enqueue Element(queue=w509, element=w507) -> (queue out=w508:refnum<queue>)  [unwired: 2 in, 2 out]
                        }
                      }
                      frame True {
                        n174 = for {
                          shift-right: [w514] -> w511
                          shift-left: w510 -> [w515]
                          tunnel: string[] ["STOP", "RESET ENCODERS", "RESET YAW", "ARDUINO MODE 0"] -> [w513] mode=indexing
                          n175 = Enqueue Element(queue=w515, element=w513) -> (queue out=w514:refnum<queue>)  [unwired: 2 in, 2 out]
                        }
                      }
                    }
                    n176 = case shown="True" w494 {
                      tunnel: [State_Type_Definitions."True Stop" ("Enum") State_Type_Definitions."True Stop" ("Enum")] -> w495
                      tunnel: [State_Type_Definitions."Idle" ("Enum") State_Type_Definitions."Idle" ("Enum")] -> w491
                      frame False {
                      }
                      frame True {
                      }
                    }
                    n177 = Select(t=w495, s=w493, f=State_Type_Definitions."Task 4_C" ("Enum")) -> (s? t:f=w499:T8)
                  }
                  frame "Exit" {
                    n178 = for {
                      shift-right: [w522] -> w519
                      shift-left: w516 -> [w523]
                      tunnel: string[] ["STOP", "RESET ENCODERS", "RESET YAW", ""] -> [w521] mode=indexing
                      n179 = Enqueue Element(queue=w523, element=w521) -> (queue out=w522:refnum<queue>)  [unwired: 2 in, 2 out]
                    }
                  }
                }
              }
            }
          }
        }
      }
      n180 = call <vilib>:"DIO Close.vi"("error in (no error)"=w7, "DIO Info In"=w10) -> ()  [unwired: 9 in, 1 out]
      n181 = call <vilib>:"DIO Close.vi"("error in (no error)"=w12, "DIO Info In"=w14) -> ()  [unwired: 9 in, 1 out]
      n182 = call <vilib>:"NavX Close.vi"("error in (no error)"=w5, "NavX Info In"=w6) -> ()  [unwired: 9 in, 1 out]
      n183 = Merge Errors "Merge Errors"(w42, w41) -> (w24:errorcluster)
      n184 = Merge Errors(w28, w24) -> (w23:errorcluster)
      n185 = Destroy User Event(user event=w45, error in=w23) -> ()  [unwired: 1 out]
      n186 = Destroy User Event(user event=w46, error in=w23) -> ()  [unwired: 1 out]
      n187 = Unregister For Events(event registration refnum=w37, error in=w23) -> ()  [unwired: 1 out]
      n188 = Release Queue(queue=w19, error in (no error)=w23) -> (error out=w4:errorcluster)  [unwired: 1 in, 2 out]
      n189 = Release Queue(queue=w36, error in (no error)=w23) -> ()  [unwired: 1 in, 3 out]
      n190 = call <vilib>:"Simple Error Handler.vi"("error in (no error)"=w4) -> ("error out"=w3:errorcluster)  [unwired: 4 in, 4 out]
      n191 = call <vilib>:"Reset myRIO.vi"("error in (no error)"=w3) -> ("error out"=→"error out":errorcluster)  [unwired: 10 in]
    }
    frame #2 {
      n192 = Wait (ms)(milliseconds to wait=u32 100) -> ()  [unwired: 1 out]
    }
  }
